vi "CODMn日志存储 (子VI).vi"(8 "流程参数":string, 9 "参数":string, 10 "日志信息":string) -> ()   [LabVIEW 2016, in "斯坦道CODMn.lvlib"]
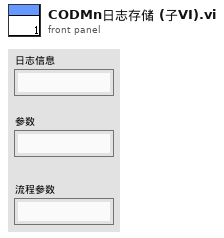
[diagram p1: front panel]
types:
  T1 = cluster{"时间标识":timestamp, "参数":string, "日志信息":string, "流程参数":string}
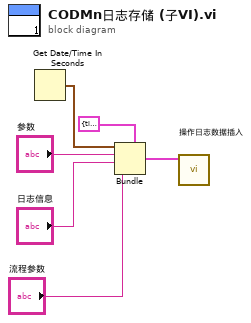
[diagram p0: block diagram]
diagram:
  n1 = Get Date/Time In Seconds() -> (seconds since 1Jan1904=w3:timestamp)
  n2 = Bundle(cluster=T1 {"时间标识"=timestamp(0 s since 1904-01-01), "参数"="", "日志信息"="", "流程参数"=""} ("data in"), "时间标识"=w3, "参数"="参数", "日志信息"="日志信息", "流程参数"="流程参数") -> (w2:T1)
  n3 = call "操作日志数据插入.vi"("data"=w2) -> ()  [unwired: 9 in, 1 out]
